vi "test-ex-date_time_string.vi"() -> ()   [LabVIEW 2012]
uses:
  <vilib>/Utility/miscctls.llb/LVDateTimeRec.ctl
panel:
  out "offset past match":i32
  out "time stamp":timestamp
  out "output string 3":string
  out "hour":dbl
  out "minutes":dbl
  out "result string 2":string
  out "seconds":dbl
  out "month":dbl
  out "result string":string
  out "day of month":dbl
  out "year":dbl
  in  "?":T1
  out "DATETIME-BOTH":dbl
  out "time string":string
  out "date string":string
  out "Date D":dbl
  out "time D":dbl
  out "variant":variant
  out "Array":dbl[](array[numeric])
  out "output string 2":string
  out "output string":string
  out "?":string
  out "?":string
  out "subarray":string[](array[string])
  in  "all rows 2":string[][](array[string])=array12547x12[150564 elements]
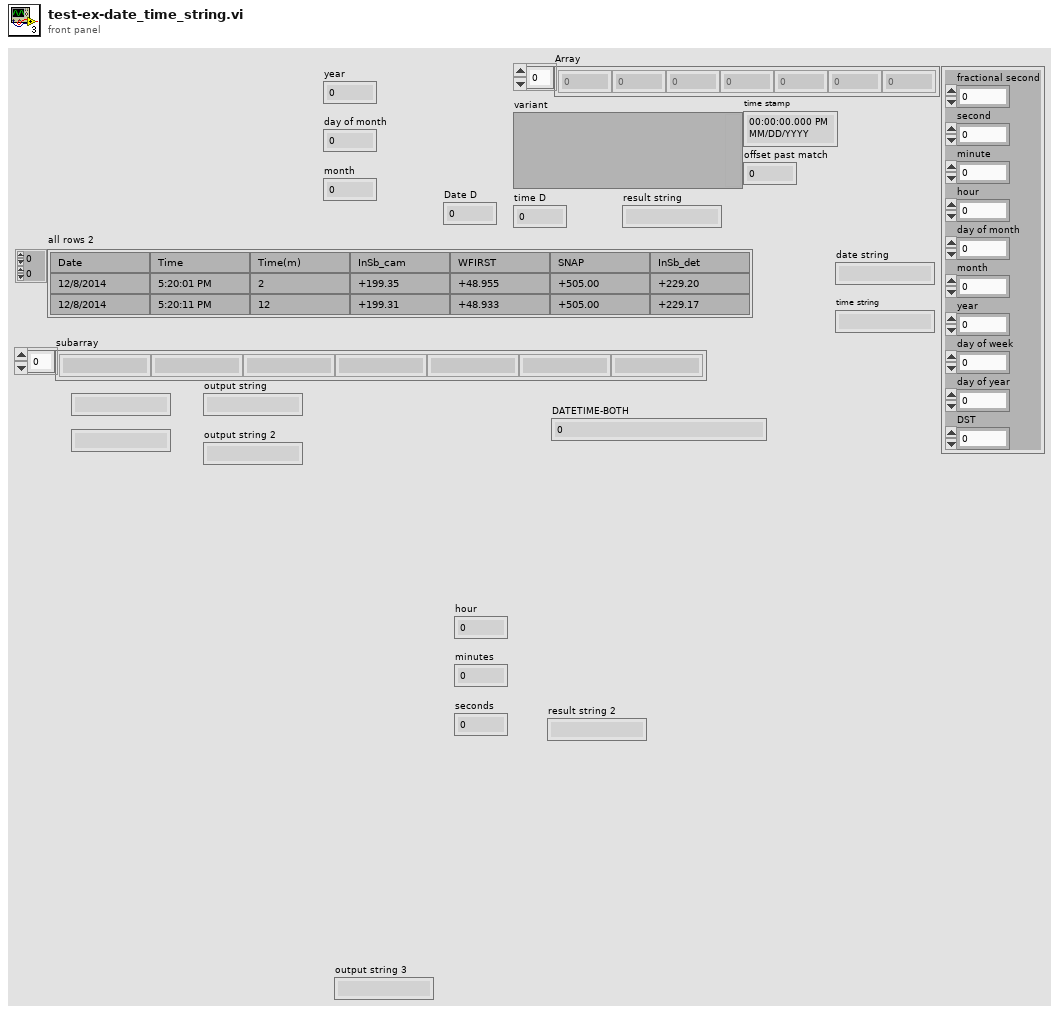
[diagram p1: front panel]
types:
  T1 = typedef "LVDateTimeRec.ctl" = cluster{"fractional second":dbl, "second":i32, "minute":i32, "hour":i32, "day of month":i32, "month":i32, "year":i32, "day of week":i32, "day of year":i32, "DST":i32}
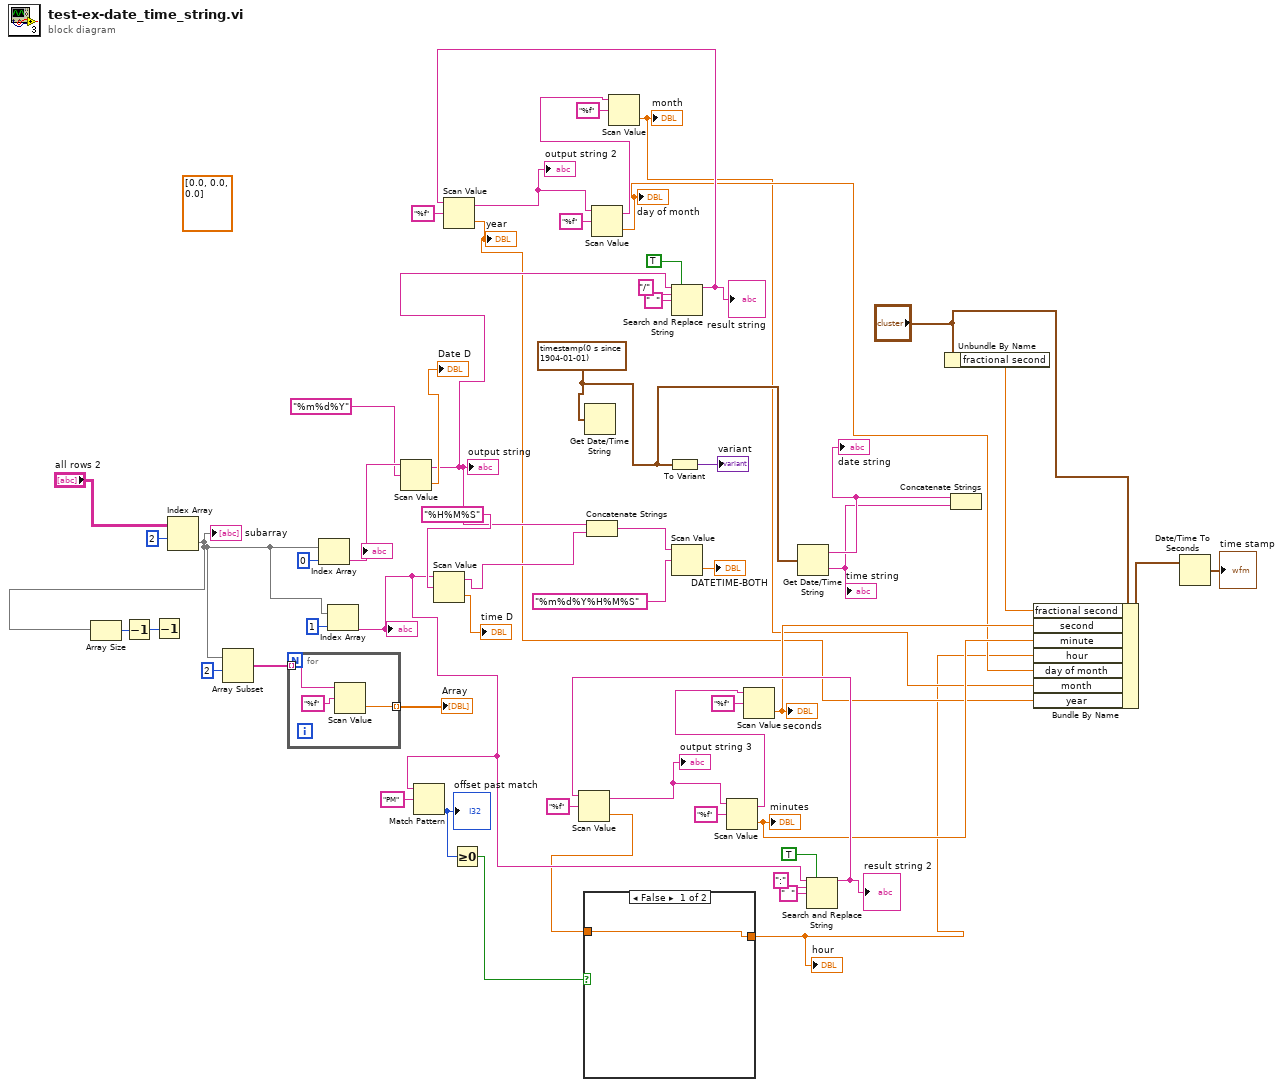
[diagram p0: block diagram]
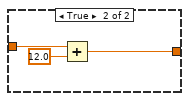
[diagram p2: hidden frame]
diagram:
  (unwired) dbl[] [0.0, 0.0, 0.0]
  w39 = timestamp(0 s since 1904-01-01)
  n1 = Index Array(array="all rows 2", index (row)=2) -> (element=w49:string[])  [unwired: 1 in]
  "subarray" <- w49
  n2 = Array Size(array=w49) -> (size(s)=w51:i32)
  n3 = Decrement(x=w51) -> (x-1=w50:i32)
  n4 = Decrement(x=w50) -> ()  [unwired: 1 out]
  n5 = Array Subset(array=w49, index=2) -> (w47:string[])  [unwired: 1 in]
  n6 = for {
    tunnel: w47 -> [w60] mode=indexing
    tunnel: [w58] -> w46 mode=indexing
    n7 = Scan Value(string=w60, format string="%f" ("string")) -> (value=w58:dbl)  [unwired: 1 in, 1 out]
  }
  "Array" <- w46
  n8 = Index Array(array=w49, index=0 ("index (row)")) -> (element=w53:string)
  "?" <- w53
  n9 = Index Array(array=w49, index=1 ("index (row)")) -> (element=w6:string)
  "?" <- w6
  n10 = Scan Value(string=w53, format string="%m%d%Y" ("string")) -> (output string=w25:string, value=→"Date D":dbl)  [unwired: 1 in]
  "output string" <- w25
  n11 = Match Pattern(string=w6, regular expression="PM") -> (offset past match=w4:i32)  [unwired: 1 in, 3 out]
  "offset past match" <- w4
  n12 = Scan Value(string=w6, format string="%H%M%S" ("string")) -> (output string=w45:string, value=→"time D":dbl)  [unwired: 1 in]
  n13 = Greater Or Equal To 0?(x=w4) -> (x >= 0?=w3:bool)
  n14 = Get Date/Time String(seconds (now)=w39) -> ()  [unwired: 2 in, 2 out]
  n15 = Concatenate Strings(w25, w45) -> (w40:string)
  n16 = To Variant(anything=w39) -> (Variant=→"variant":variant)
  n17 = Search and Replace String(replace all?=TRUE ("replace all? (F)"), input string=w25, search string="/", replace string="  " ("replace string (\"\")")) -> (result string=w24:string)  [unwired: 4 in, 3 out]
  "result string" <- w24
  n18 = Scan Value(string=w24, format string="%f") -> (output string=w29:string, value=w8:dbl)  [unwired: 1 in]
  "output string 2" <- w29
  "year" <- w8
  n19 = Scan Value(string=w29, format string="%f") -> (output string=w22:string, value=w10:dbl)  [unwired: 1 in]
  "day of month" <- w10
  n20 = Scan Value(string=w22, format string="%f") -> (value=w9:dbl)  [unwired: 1 in, 1 out]
  "month" <- w9
  n21 = Scan Value(string=w40, format string="%m%d%Y%H%M%S" ("string")) -> (value=→"DATETIME-BOTH":dbl)  [unwired: 1 in, 1 out]
  n22 = Get Date/Time String(seconds (now)=w39) -> (date string=w37:string, time string=w36:string)  [unwired: 2 in]
  "date string" <- w37
  "time string" <- w36
  n23 = Search and Replace String(replace all?=TRUE ("replace all? (F)"), input string=w6, search string=":", replace string="  " ("replace string (\"\")")) -> (result string=w19:string)  [unwired: 4 in, 3 out]
  "result string 2" <- w19
  n24 = Scan Value(string=w19, format string="%f") -> (output string=w15:string, value=w2:dbl)  [unwired: 1 in]
  "output string 3" <- w15
  n25 = case shown="False" w3 {
    tunnel: w2 -> [w61 w64]
    tunnel: [w61 w62] -> w1
    frame False {
    }
    frame True {
      n26 = Add(x=w64, y=12.0) -> (x+y=w62:dbl)
    }
  }
  "hour" <- w1
  n27 = Scan Value(string=w15, format string="%f") -> (output string=w21:string, value=w11:dbl)  [unwired: 1 in]
  "minutes" <- w11
  n28 = Scan Value(string=w21, format string="%f") -> (value=w12:dbl)  [unwired: 1 in, 1 out]
  "seconds" <- w12
  n29 = Unbundle By Name("?") -> ("fractional second"=w35:dbl)
  n30 = Concatenate Strings(w37, w36) -> ()  [unwired: 1 out]
  n31 = Bundle By Name(cluster="?", "fractional second"=w35, "second"=w12, "minute"=w11, "hour"=w1, "day of month"=w10, "month"=w9, "year"=w8) -> (w33:T1)
  n32 = Date/Time To Seconds(2:w33) -> (0:→"time stamp":timestamp)  [unwired: 1 in]
